vi "AcqType.vi"(11 "Ch & spans + mod limits":T3[](array[typedef]) {"low limit (-10V)" format="%.3f"; "high limit (10V)" format="%.3f"}) -> (0 "cDAQ i":i32[](array[numeric]), 1 "eDAQ i":i32[][](array[numeric]), 2 "cDAQ tasks":refnum<k21>[](array[refnum]), 3 "eDAQ tasks":refnum<k21>[](array[refnum]), 4 "PXI i":i32[][](array[numeric]), 5 "PXIs":refnum<k21>[](array[refnum]), 6 "O PXIs":T1[](array[typedef]))   [LabVIEW 2013]
doc: "Figures out if the channels requested are cDAQ, eDAQ or PXI and whether eDAQ channels are over multiple chassis.\n\n#optimation"
uses:
  Controls/Ch_and_Spans.ctl
  Channels_and_Index.ctl
  AcqControls/Tasks_Indices.ctl
panel:
  out "cDAQs":T2[][](array[typedef])
  out "PXIs":T2[][](array[typedef])
  out "Number of cDAQs":i32
  out "eDAQs":T2[][](array[typedef])
  out "Number of eDAQs":i32
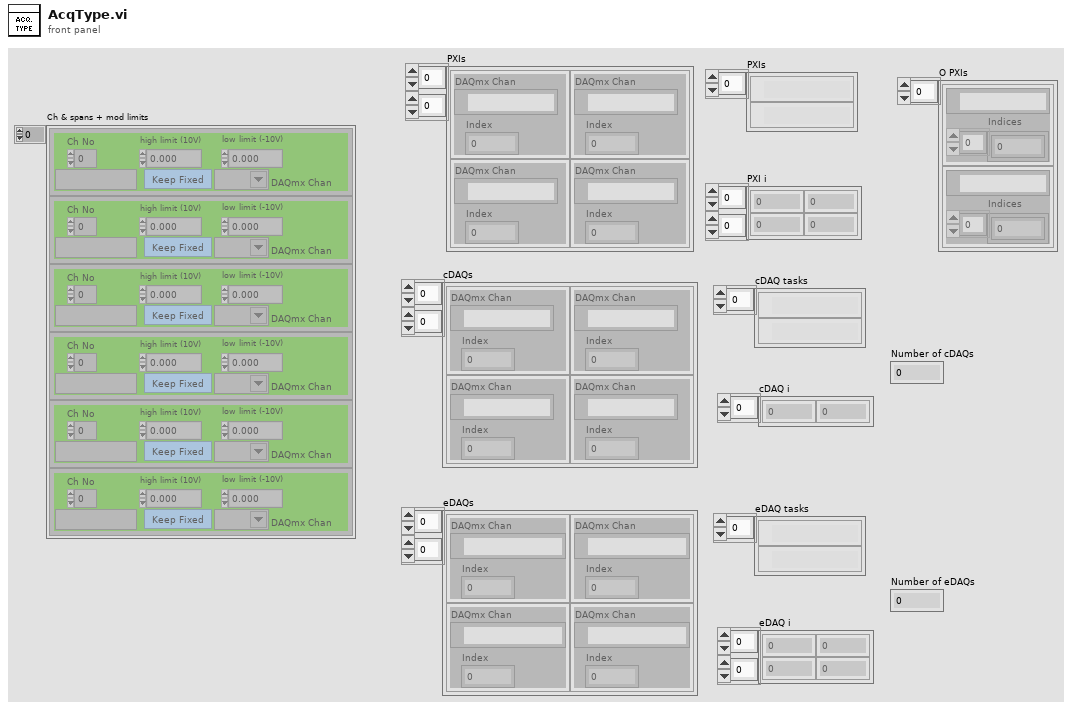
[diagram p1: front panel]
types:
  T1 = typedef "Tasks_Indices.ctl" = cluster{"task out":refnum<k21>, "Indices":i32[]}
  T2 = typedef "Channels_and_Index.ctl" = cluster{"DAQmx Chan":tag, "Index":i32}
  T3 = typedef "Ch_and_Spans.ctl" = cluster{"high limit (10V)":sgl, "low limit (-10V)":sgl, "Ch No":i16, "Var name":string, "Use Latest Calib":bool, "DAQmx Chan":tag}
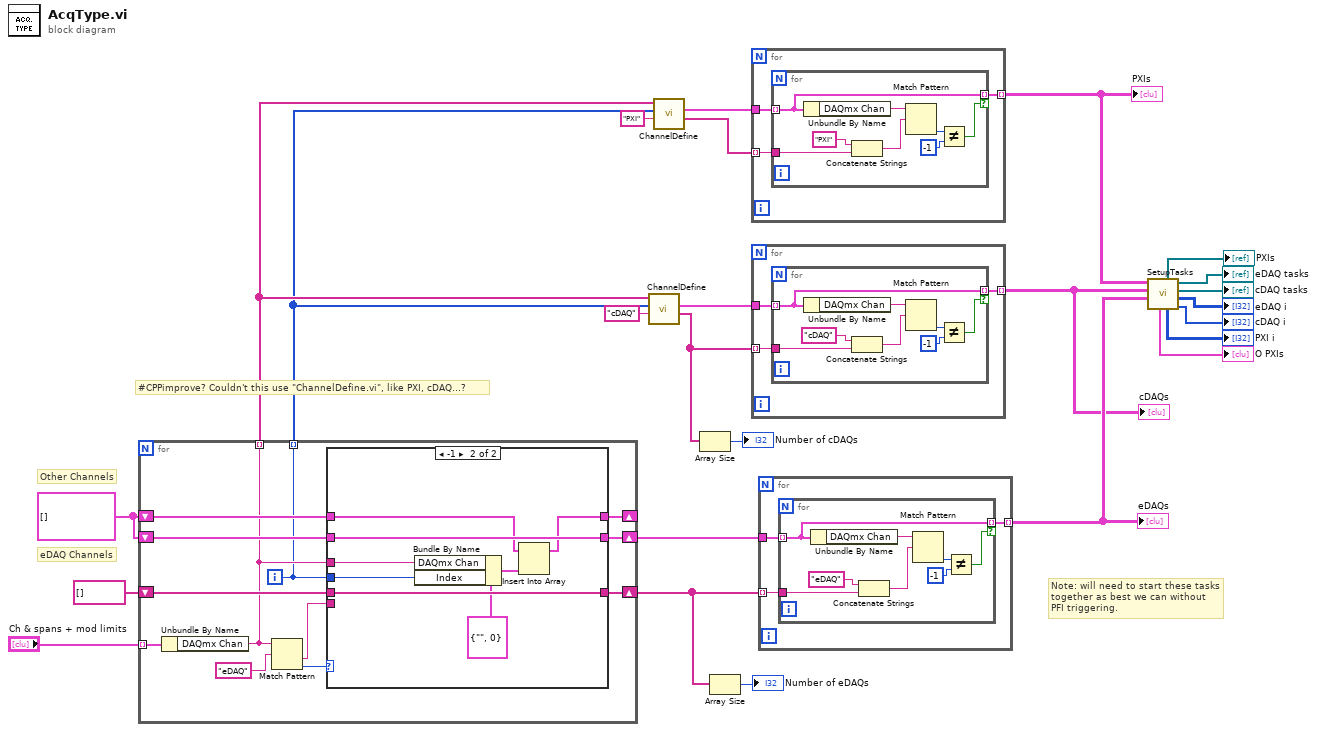
[diagram p0: block diagram]
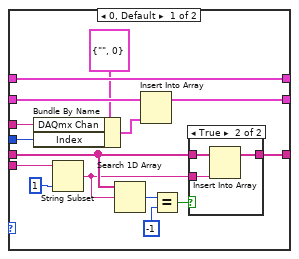
[diagram p2: hidden frame]
diagram:
  w22 = T2[] []
  # "#CPPimprove? Couldn't this use \"ChannelDefine.vi\", like PXI, cDAQ...?"
  # "Note: will need to start these tasks \ntogether as best we can without\nPFI triggering."
  # "eDAQ Channels"
  # "Other Channels"
  n1 = for {
    tunnel: "Ch & spans + mod limits" -> [w37] mode=indexing
    shift-right: [w32] -> _
    shift-left: w22 -> [w34]
    shift-right: [w31] -> w21
    shift-left: w22 -> [w33]
    shift-right: [w28] -> w20
    shift-left: string[] [] -> [w30]
    tunnel: [w27] -> w7 mode=indexing
    tunnel: [w26] -> w6 mode=indexing
    i -> [w26]
    n2 = Unbundle By Name(w37) -> ("DAQmx Chan"=w27:tag)
    n3 = Match Pattern(string=w27, regular expression="eDAQ") -> (after substring=w29:string, offset past match=w35:i32)  [unwired: 1 in, 2 out]
    n4 = case shown="-1" w35 {
      tunnel: w27 -> [w39 w58]
      tunnel: w34 -> [w52 w63]
      tunnel: w33 -> [w51 w64]
      tunnel: [w52 w62] -> w32
      tunnel: [w50 w64] -> w31
      tunnel: w30 -> [w46 w61]
      tunnel: w29 -> [w48 _]
      tunnel: [w47 w61] -> w28
      tunnel: w26 -> [w38 w57]
      frame 0, Default {
        n5 = Bundle By Name(cluster=T2 {"DAQmx Chan"="", "Index"=0} ("Indexes"), "DAQmx Chan"=w39, "Index"=w38) -> (w40:T2)
        n6 = String Subset(string=w48, length (rest)=1 ("length (rest)")) -> (substring=w45:string)  [unwired: 1 in]
        n7 = Search 1D Array(1D array=w46, element=w45) -> (index of element=w44:i32)  [unwired: 1 in]
        n8 = Insert Into Array(array=w51, new element=w40) -> (w50:T2[])  [unwired: 1 in]
        n9 = Equal?(x=w44, y=-1) -> (x = y?=w42:bool)
        n10 = case shown="True" w42 {
          tunnel: [w53 w56] -> w47
          tunnel: w46 -> [w53 w55]
          tunnel: w45 -> [_ w54]
          frame False {
          }
          frame True {
            n11 = Insert Into Array(array=w55, new element=w54) -> (w56:string[])  [unwired: 1 in]
          }
        }
      }
      frame -1 {
        n12 = Bundle By Name(cluster=T2 {"DAQmx Chan"="", "Index"=0} ("Indexes"), "DAQmx Chan"=w58, "Index"=w57) -> (w59:T2)
        n13 = Insert Into Array(array=w63, new element=w59) -> (w62:T2[])  [unwired: 1 in]
      }
    }
  }
  n14 = call "ChannelDefine.vi"("Search Term"="cDAQ", "Indices"=w6, "Tasks"=w7) -> ("Names"=w8:string[], "Tasks&Ind"=w9:T2[])  [unwired: 6 in, 1 out]
  n15 = call "ChannelDefine.vi"("Search Term"="PXI", "Indices"=w6, "Tasks"=w7) -> ("Names"=w4:string[], "Tasks&Ind"=w3:T2[])  [unwired: 6 in, 1 out]
  n16 = Array Size(array=w8) -> (size(s)=→"Number of cDAQs":i32)
  n17 = Array Size(array=w20) -> (size(s)=→"Number of eDAQs":i32)
  n18 = for {
    tunnel: w3 -> [w67]
    tunnel: w4 -> [w66] mode=indexing
    tunnel: [w65] -> w2 mode=indexing
    n19 = for {
      tunnel: w67 -> [w71] mode=indexing
      tunnel: w66 -> [w74]
      tunnel: [w71] -> w65 mode=indexing if=w69
      n20 = Unbundle By Name(w71) -> ("DAQmx Chan"=w72:tag)
      n21 = Concatenate Strings("PXI" ("regular expression"), w74) -> (w73:string)
      n22 = Match Pattern(string=w72, regular expression=w73) -> (offset past match=w70:i32)  [unwired: 1 in, 3 out]
      n23 = Not Equal?(x=w70, y=-1) -> (x != y?=w69:bool)
    }
  }
  "PXIs" <- w2
  n24 = for {
    tunnel: w9 -> [w78]
    tunnel: w8 -> [w77] mode=indexing
    tunnel: [w76] -> w15 mode=indexing
    n25 = for {
      tunnel: w78 -> [w82] mode=indexing
      tunnel: w77 -> [w85]
      tunnel: [w82] -> w76 mode=indexing if=w80
      n26 = Unbundle By Name(w82) -> ("DAQmx Chan"=w83:tag)
      n27 = Concatenate Strings("cDAQ" ("regular expression"), w85) -> (w84:string)
      n28 = Match Pattern(string=w83, regular expression=w84) -> (offset past match=w81:i32)  [unwired: 1 in, 3 out]
      n29 = Not Equal?(x=w81, y=-1) -> (x != y?=w80:bool)
    }
  }
  "cDAQs" <- w15
  n30 = for {
    tunnel: w21 -> [w89]
    tunnel: w20 -> [w88] mode=indexing
    tunnel: [w87] -> w18 mode=indexing
    n31 = for {
      tunnel: w89 -> [w93] mode=indexing
      tunnel: w88 -> [w96]
      tunnel: [w93] -> w87 mode=indexing if=w91
      n32 = Unbundle By Name(w93) -> ("DAQmx Chan"=w94:tag)
      n33 = Concatenate Strings("eDAQ" ("regular expression"), w96) -> (w95:string)
      n34 = Match Pattern(string=w94, regular expression=w95) -> (offset past match=w92:i32)  [unwired: 1 in, 3 out]
      n35 = Not Equal?(x=w92, y=-1) -> (x != y?=w91:bool)
    }
  }
  "eDAQs" <- w18
  n36 = call "SetupTasks.vi"("eDAQs"=w18, "cDAQs"=w15, "PXI"=w2) -> ("cDAQ i"=→"cDAQ i":i32[], "eDAQ i"=→"eDAQ i":i32[][], "cDAQs"=→"cDAQ tasks":refnum<k21>[], "eDAQs"=→"eDAQ tasks":refnum<k21>[], "PXI i"=→"PXI i":i32[][], "PXIs"=→"PXIs":refnum<k21>[], "O PXIs"=→"O PXIs":T1[])  [unwired: 2 in]
